vi "DesignLog.vi"(8 "error in (no error)":errorcluster, 10 "variant":variant, 11 "DesignLog":refnum<file>) -> (0 "error out":errorcluster, 2 "concatenated string":string)   [LabVIEW 2015]
uses:
  User Information.ctl
  AguaClara Library.lvlib
  Project inputs.ctl
  Basic Inputs.ctl
  Country Ring.ctl
panel:
  out "Design Inputs":T1={"Q.Plant"=0.0033333333333333335, "C.CoagDoseMax"=0.0, "C.CoagStock"=0.0, "Ti.CoagStock"=0.0, "EN.DrillSeries"=enum."English", "EN.TubeSeries"=enum."English", "N.SedTanks"=0.0, "N.SedBaysEst"=0.0, "W.SedPlate"=0.0, "L.SedPlateSheet"=0.0, "T.SedPlate"=0.0, "T.PlantWall"=0.03, "H.FlocOption"=0.01, "T.FlocBaffleRigidH"=1.7999999999999998, "T.ConcreteMin"=0.3, "T.SedWeir"=0.04, "T.FlocBaffleRigidV"=108000.0} {"T.FlocBaffleRigidV" min=0.0 max=0.2 step=0.001 format="%#.1f"; "T.SedWeir" min=0.001 max=0.2 step=0.001 format="%#.1f"; "T.SedPlate" min=0.001 max=0.05 step=0.001 format="%#.1f"; "T.FlocBaffleRigidH" min=0.0 max=0.2 step=0.001 format="%#.1f"; "T.ConcreteMin" min=0.005 max=0.2 step=0.001 format="%#.1f"; "L.SedPlateSheet" min=0.3 max=8.0 step=0.01 format="%#.1f"; "N.SedBaysEst" min=1.0 max=20.0 step=1.0 format="%#.0f"; "N.SedTanks" min=1.0 max=20.0 step=1.0 format="%#.0f"; "Ti.CoagStock" min=43200.0 max=360000.0 step=3600.0 format="%#.1f"; "H.FlocOption" min=0.5 max=4.0 step=0.01 format="%#.2f"; "C.CoagStock" min=50.0 max=500.0 step=1.0 format="%#.0f"; "C.CoagDoseMax" min=0.03 max=0.2 step=0.005 format="%#.0f"; "Q.Plant" min=0.001 max=0.2 step=0.0001 format="%#.1f"; "T.PlantWall" min=0.05 max=0.5 step=0.001 format="%#.1f"; "W.SedPlate" min=0.5 max=3.0 step=0.001 format="%#.1f"}
  out "Project inputs":T2
  out "User Information":T3 {"Country" items=["Afghanistan", "Aland Islands", "Albania", "Algeria", "American Samoa", "Andorra", "Angola", "Anguilla", "Antarctica", "Antigua And Barbuda", "Argentina", "Armenia", "Aruba", "Australia", "Austria", "Azerbaijan", "Bahamas", "Bahrain", "Bangladesh", "Barbados", "Belarus", "Belgium", "Belize", "Benin", "Bermuda", "Bhutan", "Bolivia", "Bosnia And Herzegovina", "Botswana", "Bouvet Island", "Brazil", "British Indian Ocean Territory", "Brunei Darussalam", "Bulgaria", "Burkina Faso", "Burundi", "Cambodia", "Cameroon", "Canada", "Cape Verde", "Cayman Islands", "Central African Republic", "Chad", "Chile", "China", "Christmas Island", "Cocos (Keeling) Islands", "Colombia", "Comoros", "Congo", "Congo, The Democratic Republic Of The", "Cook Islands", "Costa Rica", "Cote D'Ivoire", "Croatia", "Cuba", "Cyprus", "Czech Republic", "Denmark", "Djibouti", "Dominica", "Dominican Republic", "Ecuador", "Egypt", "El Salvador", "Equatorial Guinea", "Eritrea", "Estonia", "Ethiopia", "Falkland Islands (Malvinas)", "Faroe Islands", "Fiji", "Finland", "France", "French Guiana", "French Polynesia", "French Southern Territories", "Gabon", "Gambia", "Georgia", "Germany", "Ghana", "Gibraltar", "Greece", "Greenland", "Grenada", "Guadeloupe", "Guam", "Guatemala", "Guernsey", "Guinea", "Guinea-Bissau", "Guyana", "Haiti", "Heard Island And Mcdonald Islands", "Holy See (Vatican City State)", "Honduras", "Hong Kong", "Hungary", "Iceland", "India", "Indonesia", "Iran, Islamic Republic Of", "Iraq", "Ireland", "Isle Of Man", "Israel", "Italy", "Jamaica", "Japan", "Jersey", "Jordan", "Kazakhstan", "Kenya", "Kiribati", "Korea, Democratic People'S Republic Of", "Korea, Republic Of", "Kuwait", "Kyrgyzstan", "Lao People'S Democratic Republic", "Latvia", "Lebanon", "Lesotho", "Liberia", "Libyan Arab Jamahiriya", "Liechtenstein", "Lithuania", "Luxembourg", "Macao", "Macedonia, The Former Yugoslav Republic Of", "Madagascar", "Malawi", "Malaysia", "Maldives", "Mali", "Malta", "Marshall Islands", "Martinique", "Mauritania", "Mauritius", "Mayotte", "Mexico", "Micronesia, Federated States Of", "Moldova, Republic Of", "Monaco", "Mongolia", "Montserrat", "Morocco", "Mozambique", "Myanmar", "Namibia", "Nauru", "Nepal", "Netherlands", "Netherlands Antilles", "New Caledonia", "New Zealand", "Nicaragua", "Niger", "Nigeria", "Niue", "Norfolk Island", "Northern Mariana Islands", "Norway", "Oman", "Pakistan", "Palau", "Palestinian Territory, Occupied", "Panama", "Papua New Guinea", "Paraguay", "Peru", "Philippines", "Pitcairn", "Poland", "Portugal", "Puerto Rico", "Qatar", "Reunion", "Romania", "Russian Federation", "Rwanda", "Saint Helena", "Saint Kitts And Nevis", "Saint Lucia", "Saint Pierre And Miquelon", "Saint Vincent And The Grenadines", "Samoa", "San Marino", "Sao Tome And Principe", "Saudi Arabia", "Senegal", "Serbia And Montenegro", "Seychelles", "Sierra Leone", "Singapore", "Slovakia", "Slovenia", "Solomon Islands", "Somalia", "South Africa", "South Georgia And The South Sandwich Islands", "Spain", "Sri Lanka", "Sudan", "Suriname", "Svalbard And Jan Mayen", "Swaziland", "Sweden", "Switzerland", "Syrian Arab Republic", "Taiwan, Province Of China", "Tajikistan", "Tanzania, United Republic Of", "Thailand", "Timor-Leste", "Togo", "Tokelau", "Tonga", "Trinidad And Tobago", "Tunisia", "Turkey", "Turkmenistan", "Turks And Caicos Islands", "Tuvalu", "Uganda", "Ukraine", "United Arab Emirates", "United Kingdom", "United States", "United States Minor Outlying Islands", "Uruguay", "Uzbekistan", "Vanuatu", "Venezuela", "Viet Nam", "Virgin Islands, British", "Virgin Islands, U.S.", "Wallis And Futuna", "Western Sahara", "Yemen", "Zambia", "Zimbabwe", "(Not Specified)"]}
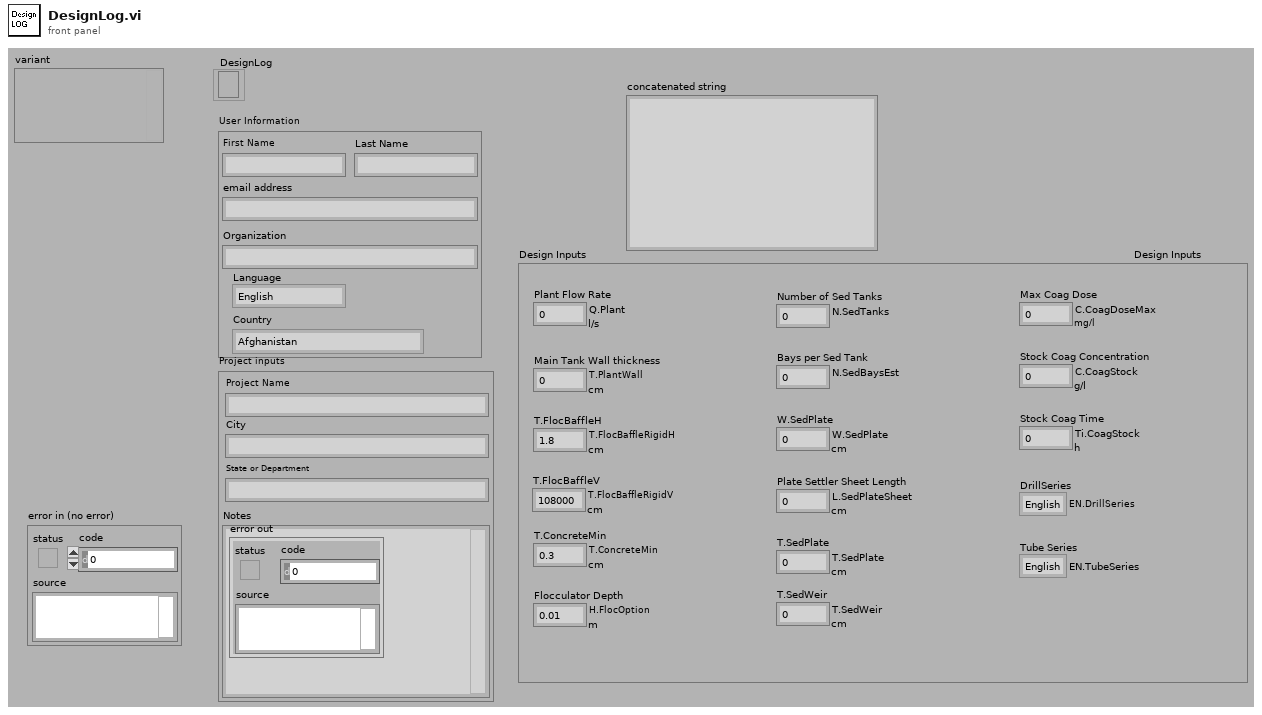
[diagram p1: front panel]
types:
  T1 = typedef "AguaClara Library.lvlib/Basic Inputs.ctl" = cluster{"Q.Plant":dbl[unit], "C.CoagDoseMax":dbl[unit], "C.CoagStock":dbl[unit], "Ti.CoagStock":dbl[unit], "EN.DrillSeries":enum16{"English", "Metric"}, "EN.TubeSeries":enum16{"English", "Metric"}, "N.SedTanks":dbl, "N.SedBaysEst":dbl, "W.SedPlate":dbl[unit], "L.SedPlateSheet":dbl[unit], "T.SedPlate":dbl[unit], "T.PlantWall":dbl[unit], "H.FlocOption":dbl[unit], "T.FlocBaffleRigidH":dbl[unit], "T.ConcreteMin":dbl[unit], "T.SedWeir":dbl[unit], "T.FlocBaffleRigidV":dbl[unit]}
  T2 = typedef "AguaClara Library.lvlib/Project inputs.ctl" = cluster{"Project Name":string, "City":string, "State":string, "Notes":string}
  T3 = typedef "AguaClara Library.lvlib/User Information.ctl" = cluster{"First Name":string, "Last Name":string, "Email Address":string, "Organization":string, "Language":enum16{"English", "Español", "French"}, "Country":T4}
  T4 = typedef "Country Ring.ctl" = u16
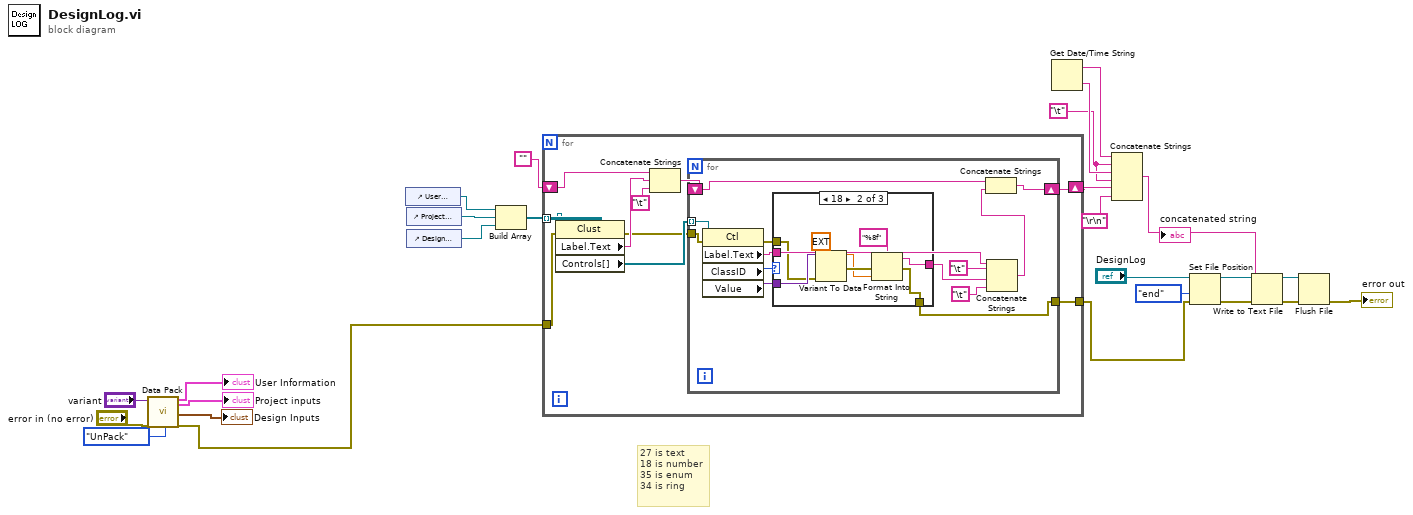
[diagram p0: block diagram]
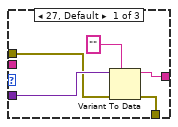
[diagram p2: hidden frame]
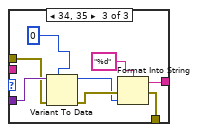
[diagram p3: hidden frame]
diagram:
  w10 = "\t"
  # "27 is text\n18 is number\n35 is enum\n34 is ring"
  n1 = call "Data Pack.vi"("error in"="error in (no error)", "Packed In"="variant", "Data transform"=enum16{"Pack", "UnPack"}."UnPack") -> ("User Information out"=→"User Information":T3, "Project Info out"=→"Project inputs":T2, "Design Inputs out"=→"Design Inputs":T1, "error out"=w13:errorcluster)  [unwired: 9 in, 4 out]
  n2 = control-ref of="User Information"() -> (w26:refnum<vi>)
  n3 = control-ref of="Project inputs"() -> (w25:refnum<vi>)
  n4 = control-ref of="Design Inputs"() -> (w24:refnum<vi>)
  n5 = Build Array(w26, w25, w24) -> (w23:refnum<vi>[])
  n6 = for {
    tunnel: w23 -> [w36] mode=indexing
    shift-right: [w31] -> w21
    shift-left: "" -> [w30]
    tunnel: w13 -> [w29]
    tunnel: [w27] -> w2
    n7 = property class="Clust"(reference=w36, error in=w29) -> (error out=w28:errorcluster, "Label.Text"=w33:string, "Controls[]"=w35:refnum<vi>[])  [unwired: 1 out]
    n8 = Concatenate Strings(w30, w33, "\t") -> (w34:string)
    n9 = for {
      tunnel: w35 -> [w49] mode=indexing
      shift-right: [w43] -> w31
      shift-left: w34 -> [w40]
      tunnel: w28 -> [w39]
      tunnel: [w37] -> w27
      n10 = property class="Ctl"(reference=w49, error in=w39) -> (error out=w38:errorcluster, "Label.Text"=w47:string, "ClassID"=w41:u32, "Value"=w48:variant)  [unwired: 1 out]
      n11 = case shown="18" w41 {
        tunnel: w48 -> [w54 w62 w70]
        tunnel: w47 -> [_ _ _]
        tunnel: [w53 w57 w69] -> w46
        tunnel: w38 -> [w51 w56 w64]
        tunnel: [w50 w55 w63] -> w37
        frame 27, Default {
          n12 = Variant To Data(error in=w51, type="", Variant=w54) -> (data=w53:string, error out=w50:errorcluster)
        }
        frame 18 {
          n13 = Variant To Data(error in=w56, type=ext 0.0, Variant=w62) -> (data=w59:ext, error out=w60:errorcluster)
          n14 = Format Into String(format string="%8f", error in=w60, w59) -> (resulting string=w57:string, error out=w55:errorcluster)  [unwired: 1 in]
        }
        frame 34, 35 {
          n15 = Variant To Data(error in=w64, type=0, Variant=w70) -> (data=w65:i32, error out=w67:errorcluster)
          n16 = Format Into String(format string="%d", error in=w67, w65) -> (resulting string=w69:string, error out=w63:errorcluster)  [unwired: 1 in]
        }
      }
      n17 = Concatenate Strings(w47, "\t", w46, "\t") -> (w42:string)
      n18 = Concatenate Strings(w40, w42) -> (w43:string)
    }
  }
  n19 = Get Date/Time String() -> (date string=w11:string, time string=w12:string)  [unwired: 3 in]
  n20 = Concatenate Strings(w11, w10, w12, w10, w21, "\r\n") -> (w19:string)
  "concatenated string" <- w19
  n21 = Set File Position(refnum="DesignLog", from (0:start)=enum16{"start", "end", "current"}."end", error in=w2) -> (refnum out=w3:refnum<file>, error out=w1:errorcluster)  [unwired: 1 in]
  n22 = Write to Text File(file (use dialog)=w3, text=w19, error in=w1) -> (refnum out=w9:refnum<file>, error out=w8:errorcluster)  [unwired: 1 in, 1 out]
  n23 = Flush File(refnum=w9, error in=w8) -> (error out=→"error out":errorcluster)  [unwired: 1 out]
